vi "Configure Lookup Table.vi"(0 "Instrument Handle In":refnum<k21>, 1 "Selector String":string, 5 "Lookup Table Configuration":T1={"Type"=1, "Correction Type"=0, "Threshold Enabled"=1, "Threshold Type"=0, "Threshold Level (dB or dBm)"=-20.0, "Step Size (dB)"=0.1} {"Type" items=["Log", "Linear"]; "Correction Type" items=["Magnitude and Phase", "Magnitude Only", "Phase Only"]; "Threshold Level (dB or dBm)" format="%.2g"; "Threshold Type" items=["Relative", "Absolute"]; "Threshold Enabled" items=["False", "True"]}, 11 "error in (no error)":errorcluster) -> (4 "Instrument Handle Out":refnum<k21>, 15 "error out":errorcluster)   [LabVIEW 2019, in "RFmxDPD.lvlib"]
doc: "Configures common settings for lookup table based DPD."
uses:
  RFmxDPD.lvlib
  Typedefs/Lookup Table Configuration.ctl
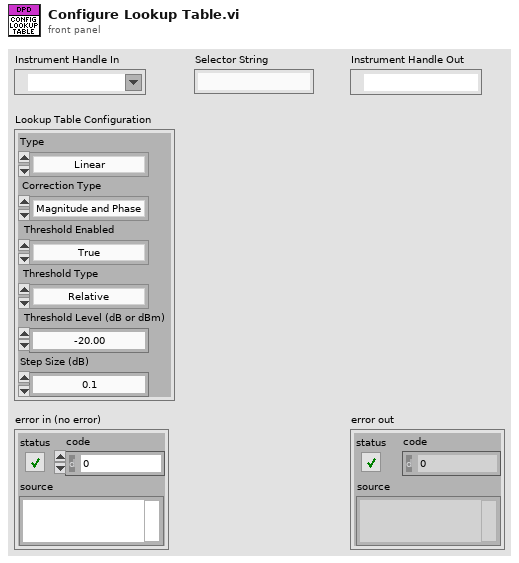
[diagram p1: front panel]
types:
  T1 = typedef "RFmxDPD.lvlib/Lookup Table Configuration.ctl" = cluster{"Type":i32, "Correction Type":i32, "Threshold Enabled":i32, "Threshold Type":i32, "Threshold Level (dB or dBm)":dbl, "Step Size (dB)":dbl}
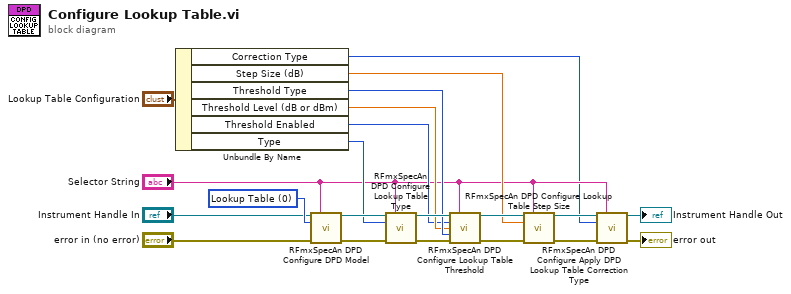
[diagram p0: block diagram]
diagram:
  w21 = 0 items=["Lookup Table", "Memory Polynomial", "Generalized Memory Polynomial"] ("DPD Model")
  n1 = Unbundle By Name("Lookup Table Configuration") -> ("Correction Type"=w3:i32, "Step Size (dB)"=w12:dbl, "Threshold Type"=w11:i32, "Threshold Level (dB or dBm)"=w10:dbl, "Threshold Enabled"=w9:i32, "Type"=w8:i32)
  n2 = call <vilib>:"RFmxSpecAn DPD Configure DPD Model.vi"("Instrument Handle In"="Instrument Handle In", "Selector String"="Selector String", "DPD Model"=w21, "error in (no error)"="error in (no error)") -> ("Instrument Handle Out"=w16:refnum<k21>, "error out"=w15:errorcluster)  [unwired: 10 in]
  n3 = call <vilib>:"RFmxSpecAn DPD Configure Lookup Table Type.vi"("Instrument Handle In"=w16, "Selector String"="Selector String", "DPD LUT Type"=w8, "error in (no error)"=w15) -> ("Instrument Handle Out"=w14:refnum<k21>, "error out"=w13:errorcluster)  [unwired: 10 in]
  n4 = call <vilib>:"RFmxSpecAn DPD Configure Lookup Table Threshold.vi"("Instrument Handle In"=w14, "Selector String"="Selector String", "Threshold Enabled"=w9, "Threshold Level (dB or dBm)"=w10, "Threshold Type"=w11, "error in (no error)"=w13) -> ("Instrument Handle Out"=w20:refnum<k21>, "error out"=w19:errorcluster)  [unwired: 8 in]
  n5 = call <vilib>:"RFmxSpecAn DPD Configure Lookup Table Step Size.vi"("Instrument Handle In"=w20, "Selector String"="Selector String", "Step Size (dB)"=w12, "error in (no error)"=w19) -> ("Instrument Handle Out"=w6:refnum<k21>, "error out"=w5:errorcluster)  [unwired: 10 in]
  n6 = call <vilib>:"RFmxSpecAn DPD Configure Apply DPD Lookup Table Correction Type.vi"("Instrument Handle In"=w6, "Selector String"="Selector String", "LUT Correction Type"=w3, "error in (no error)"=w5) -> ("Instrument Handle Out"=→"Instrument Handle Out":refnum<k21>, "error out"=→"error out":errorcluster)  [unwired: 10 in]
